vi "Untitled 1 (SubVI).vi"(8 "error in":errorcluster, 11 "output cluster":T1) -> (0 "error out":errorcluster, 3 "Array":dbl[][](array[numeric]))   [LabVIEW 2009]
uses:
  Type Def/xijk_cluster.ctl
panel:
  out "Array 3":dbl[][](array[numeric])
  out "Array 2":dbl[][](array[numeric])
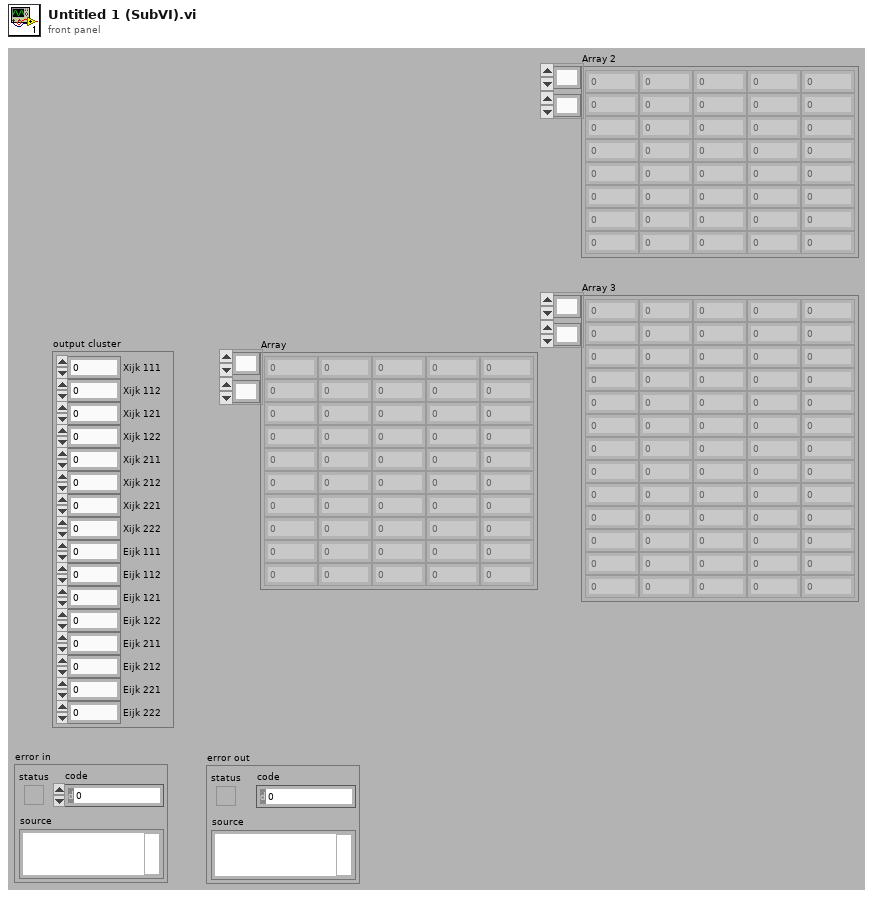
[diagram p1: front panel]
types:
  T1 = typedef "xijk_cluster.ctl" = cluster{"Xijk 111":sgl, "Xijk 112":sgl, "Xijk 121":sgl, "Xijk 122":sgl, "Xijk 211":sgl, "Xijk 212":sgl, "Xijk 221":sgl, "Xijk 222":sgl, "Eijk 111":sgl, "Eijk 112":sgl, "Eijk 121":sgl, "Eijk 122":sgl, "Eijk 211":sgl, "Eijk 212":sgl, "Eijk 221":sgl, "Eijk 222":sgl}
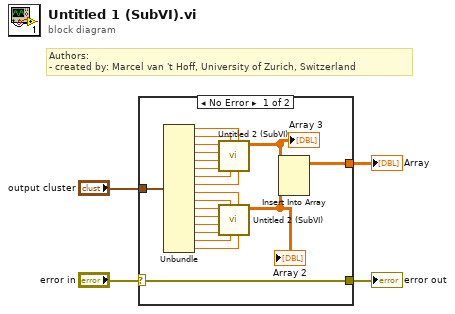
[diagram p0: block diagram]
diagram:
  # "Authors: \n- created by: Marcel van 't Hoff, University of Zurich, Switzerland"
  n1 = case shown="No Error" "error in" {
    selector: "error in" -> [w5 w26]
    tunnel: "output cluster" -> [w19 _]
    tunnel: [w6 _] -> w3
    tunnel: [w5 w26] -> w1
    frame #0 {
      n2 = Unbundle(w19) -> ("Xijk 111"=w18:sgl, "Xijk 112"=w20:sgl, "Xijk 121"=w21:sgl, "Xijk 122"=w23:sgl, "Xijk 211"=w22:sgl, "Xijk 212"=w24:sgl, "Xijk 221"=w25:sgl, "Xijk 222"=w17:sgl, "Eijk 111"=w16:sgl, "Eijk 112"=w15:sgl, "Eijk 121"=w14:sgl, "Eijk 122"=w13:sgl, "Eijk 211"=w12:sgl, "Eijk 212"=w11:sgl, "Eijk 221"=w10:sgl, "Eijk 222"=w9:sgl)
      n3 = call "Untitled 2 (SubVI).vi"("222"=w17, "111"=w18, "221"=w25, "112"=w20, "212"=w24, "211"=w22, "122"=w23, "121"=w21) -> ("Array"=w8:dbl[][])  [unwired: 3 in]
      "Array 3" <- w8
      n4 = call "Untitled 2 (SubVI).vi"("222"=w9, "111"=w16, "221"=w10, "112"=w15, "212"=w11, "211"=w12, "122"=w13, "121"=w14) -> ("Array"=w7:dbl[][])  [unwired: 3 in]
      "Array 2" <- w7
      n5 = Insert Into Array(array=w8, new element=w7) -> (w6:dbl[][])  [unwired: 2 in]
    }
    frame #1 {
    }
  }
  "Array" <- w3
  "error out" <- w1
